vi "Check Data Buffer.vi"(8 "error in (no error)":errorcluster, 11 "UART Actor in":refnum<class "UART Actor.lvclass">) -> (0 "error out":errorcluster, 3 "UART Actor out":refnum<class "UART Actor.lvclass">)   [LabVIEW 2020, in "UART Actor.lvlib" / "UART Actor.lvclass"]
uses:
  UART Actor.lvclass
  UART Actor.lvclass/UART Actor.ctl
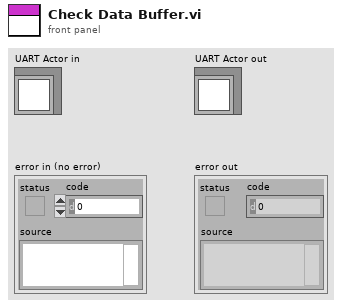
[diagram p1: front panel]
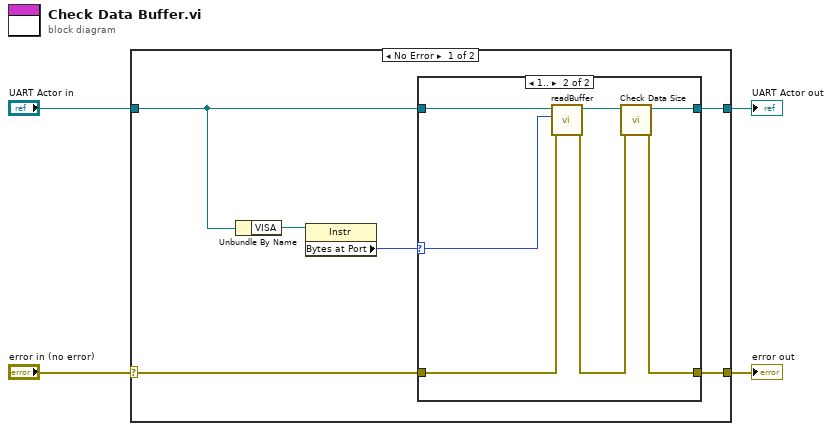
[diagram p0: block diagram]
diagram:
  n1 = case shown="No Error" "error in (no error)" {
    selector: "error in (no error)" -> [w7 w21]
    tunnel: [w6 w21] -> w3
    tunnel: [w9 w20] -> w1
    tunnel: "UART Actor in" -> [w8 w20]
    frame No Error {
      n2 = Unbundle By Name(w8) -> ("VISA"=w10:refnum<visa-resource-name>)
      n3 = property class="Instr"(reference=w10) -> ("Bytes at Port"=w5:u32)  [unwired: 1 in, 2 out]
      n4 = case shown="1.." w5 {
        selector: w5 -> [_ w17]
        tunnel: [w12 w15] -> w9
        tunnel: w8 -> [w12 w19]
        tunnel: w7 -> [w11 w18]
        tunnel: [w11 w13] -> w6
        frame 0, Default {
        }
        frame 1.. {
          n5 = call "readBuffer.vi"("error in (no error)"=w18, "byte count"=w17, "UART Actor in"=w19) -> ("error out"=w14:errorcluster, "UART Actor out"=w16:refnum<class "UART Actor.lvclass">)  [unwired: 7 in]
          n6 = call "Check Data Size.vi"("error in (no error)"=w14, "UART Actor in"=w16) -> ("error out"=w13:errorcluster, "UART Actor out"=w15:refnum<class "UART Actor.lvclass">)  [unwired: 8 in]
        }
      }
    }
    frame Error {
    }
  }
  "error out" <- w3
  "UART Actor out" <- w1
